vi "Configure_PSG_ Frequency.vi"(1 "Frequency [GHz]":dbl=100000.0, 2 "VISA resource name":refnum<visa-resource-name>) -> ()   [LabVIEW 2011]
doc: "This example shows how to configure the frequency and power of the output signal."
uses:
  <vilib>/Utility/error.llb/DialogType.ctl
  <instrlib>/Agilent PSG MXG Series/Agilent PSG MXG Series.lvlib
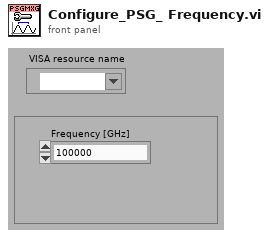
[diagram p1: front panel]
types:
  T1 = typedef "DialogType.ctl" = u16
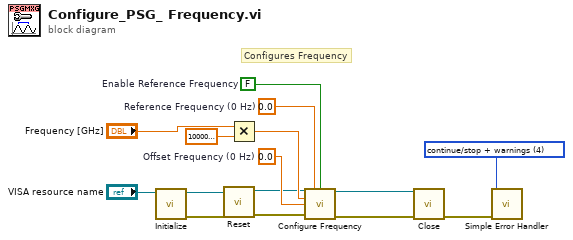
[diagram p0: block diagram]
diagram:
  w3 = T1 4 items=["no dialog", "OK message", "continue or stop message", "OK message + warnings", "continue/stop + warnings"] ("type of dialog (OK msg:1)")
  w11 = 0.0  # Offset Frequency (0 Hz)
  w12 = 0.0  # Reference Frequency (0 Hz)
  w13 = FALSE  # Enable Reference Frequency
  # "Configures Frequency"
  n1 = call <instrlib>:"Initialize.vi"("VISA resource name"="VISA resource name") -> ("error out"=w5:errorcluster, "VISA resource name out"=w7:refnum<visa-resource-name>)  [unwired: 9 in]
  n2 = call <instrlib>:"Reset.vi"("error in (no error)"=w5, "VISA resource name"=w7) -> ("error out"=w4:errorcluster, "VISA resource name out"=w6:refnum<visa-resource-name>)  [unwired: 8 in]
  n3 = Multiply(x="Frequency [GHz]", y=1000000000.0) -> (x*y=w8:dbl)
  n4 = call <instrlib>:"Configure Frequency.vi"("VISA resource name"=w6, "Reference Frequency (0 Hz)"=w12, "Enable Reference Frequency (F:Disable)"=w13, "Frequency (100 kHz)"=w8, "Offset Frequency (0 Hz)"=w11, "error in (no error)"=w4) -> ("VISA resource name out"=w2:refnum<visa-resource-name>, "error out"=w1:errorcluster)  [unwired: 8 in]
  n5 = call <instrlib>:"Close.vi"("error in (no error)"=w1, "VISA resource name"=w2) -> ("error out"=w15:errorcluster)  [unwired: 9 in]
  n6 = call <vilib>:"Simple Error Handler.vi"("type of dialog (OK msg:1)"=w3, "error in (no error)"=w15) -> ()  [unwired: 3 in, 5 out]
